vi "NMR10.vi"() -> ()   [LabVIEW 2013]
uses:
  <vilib>/Analysis/NI_AALBase.lvlib
panel:
  in  "Amp of Q curve":dbl=16.5 format="%_3f"
  in  "Subtract Q curve":bool=TRUE
  in  "Adjust Tune":bool=TRUE
  out "IF Offset":dbl(graph)=3.131691772460936
  out "Pedestal Difference":dbl(graph)=0.04542741927075716
  out "# Good Spectra":i32=99
  in  "Quality cuts":bool=TRUE
  out "Pedestal OK":bool=TRUE
  out "Sweep #":i32=2
  out "1st Sweep":bool
  out "ADC voltages OK":bool=TRUE
  out "Peak Height Distribution":cluster{"Y":dbl[], "Y":dbl[]}[](graph)=[{"Y"=[0.2355519843953429, 0.23617339654540798, 0.2367948086954731, 0.2374162208455382, 0.2380376329956033, 0.2386590451456684, 0.23928045729573352, 0.2399018694457986, 0.24052328159586372, 0.2411446937459288, 0.24176610589599393, 0.24238751804605904, 0.24300893019612413, 0.24363034234618924, 0.24425175449625433, 0.24487316664631945, 0.24549457879638456, 0.24611599094644965, 0.24673740309651476, 0.24735881524657988, 0.24798022739664496, 0.24860163954671008, 0.24922305169677517, 0.24984446384684028, 0.2504658759969054, 0.2510872881469705, 0.25170870029703557, 0.2523301124471007, 0.2529515245971658, 0.2535729367472309, 0.25419434889729603, 0.25481576104736114, 0.2554371731974262, 0.2560585853474913, 0.25667999749755643, 0.25730140964762155, 0.25792282179768666, 0.2585442339477517, 0.25916564609781684, 0.25978705824788195, 0.26040847039794707, 0.2610298825480122, 0.26165129469807724, 0.26227270684814236, 0.26289411899820747, 0.2635155311482726, 0.2641369432983377, 0.26475835544840276, 0.2653797675984679, 0.266001179748533, 0.2666225918985981, 0.2672440040486632, 0.26786541619872833, 0.2684868283487934, 0.2691082404988585, 0.2697296526489236, 0.27035106479898874, 0.27097247694905385, 0.2715938890991189, 0.272215301249184, 0.27283671339924914, 0.27345812554931426, 0.27407953769937937, 0.27470094984944443, 0.27532236199950955, 0.27594377414957466, 0.2765651862996398, 0.2771865984497049, 0.27780801059976995, 0.27842942274983506, 0.2790508348999002, 0.2796722470499653, 0.2802936592000304, 0.2809150713500955, 0.2815364835001606, 0.2821578956502257, 0.2827793078002908, 0.28340071995035593, 0.28402213210042104, 0.2846435442504861, 0.2852649564005512, 0.28588636855061633, 0.28650778070068145, 0.28712919285074656, 0.2877506050008116, 0.28837201715087674, 0.28899342930094185, 0.28961484145100697, 0.2902362536010721, 0.29085766575113714, 0.29147907790120225, 0.29210049005126737, 0.2927219022013325, 0.2933433143513976, 0.2939647265014627, 0.2945861386515278, 0.2952075508015929, 0.295828962951658, 0.2964503751017231, 0.29707178725178823], "Y"=[1.0, 0.0, 0.0, 0.0, 0.0, 0.0, 0.0, 0.0, 0.0, 0.0, 0.0, 1.0, 0.0, 0.0, 1.0, 0.0, 0.0, 0.0, 0.0, 0.0, 0.0, 0.0, 1.0, 1.0, 0.0, 1.0, 1.0, 2.0, 0.0, 1.0, 3.0, 1.0, 1.0, 0.0, 3.0, 2.0, 2.0, 2.0, 3.0, 2.0, 0.0, 4.0, 1.0, 1.0, 4.0, 3.0, 3.0, 2.0, 4.0, 0.0, 4.0, 2.0, 3.0, 1.0, 1.0, 2.0, 4.0, 4.0, 3.0, 0.0, 3.0, 4.0, 2.0, 2.0, 1.0, 2.0, 0.0, 1.0, 0.0, 0.0, 1.0, 2.0, 0.0, 0.0, 1.0, 1.0, 1.0, 0.0, 0.0, 1.0, 0.0, 0.0, 0.0, 0.0, 0.0, 1.0, 0.0, 0.0, 0.0, 0.0, 0.0, 0.0, 0.0, 0.0, 0.0, 0.0, 0.0, 0.0, 0.0, 1.0]}]
  in  "# of Sweeps":i32=100
  out "Std Dev (V)":dbl=0.009965193633611454 format="%_2g"
  out "Peak mean (V)":dbl=0.2655884316981644 format="%_4g"
  out "Peak Height":dbl(graph)=0.26806171289062286
  in  "Raw Data":bool
  in  "Tank RF ON":bool=TRUE
  in  "IF Atten (dB)":i8 min=0 max=35 step=5
  in  "IFoffset (V)":dbl=3.131691772460936 min=0.0 max=3000.0 step=0.001 format="%.3f"
  in  "Tune  (V)":dbl=1.5059999999999982 min=0.0 max=5.0 step=0.001 format="%.3f"
  in  "Hi / Lo Gain":bool
  out "Voltage Array":sgl[](array[numeric])=[0.39486083, 0.39415282, 0.37740478, 0.36463624, 0.35776368, 0.33198243, 0.3107544, 0.32425538, 0.2953125, 0.27941895, 0.2874756, 0.2617798, 0.2520508, 0.24379882, 0.24141845, 0.22194824, 0.19313964, 0.1977295, 0.19276123, 0.17390136, 0.17283936, 0.16755371, 0.14387207, 0.12849121, 0.12796631, 0.13111572, 0.1216919, 0.10755615, 0.08287354, 0.06949463, 0.07113037, 0.062060546, 0.036108397, 0.032678224, 0.013000488, 0.0095825195, 0.01607666, 0.0040771486, 0.005566406, -0.01229248, 0.0024536133, -0.0022338866, -0.017175293, -0.029064942, -0.02878418, -0.05206299, -0.04116211, -0.05924072, -0.060913086, -0.07078858, -0.06147461, -0.0708252, -0.09482422, -0.09287109, -0.08811035, -0.10527344, -0.10979004, -0.09885254, -0.10852051, -0.12213135, -0.12347412, -0.13558349, -0.13809815, -0.1430664, -0.16062012, -0.16202393, -0.16688232, -0.1687622, -0.1630371, -0.17376709, -0.19066162, -0.17672119, -0.19134521, -0.19102784, -0.20743409, -0.1963379, -0.19866943, -0.20877686, -0.2253662, -0.21699218, -0.22194824, -0.22015381, -0.22921142, -0.21680908, -0.21575928, -0.23323974, -0.21798095, -0.22463378, -0.23702392, -0.21989746, -0.22541504, -0.20744629, -0.202063, -0.19719239, -0.18527833, -0.18197021, -0.13729247, -0.11975098, -0.061206054, -0.022375489, 0.010229493, 0.036230467, -0.003857422, -0.054382324, -0.0927124, -0.12541504, -0.1385376, -0.15421143, -0.16003418, -0.15662841, -0.19451904, -0.18380126, -0.19353028, -0.19848633, -0.19445801, -0.21176758, -0.20693359, -0.19925538, -0.19172363, -0.18999024, -0.19869384, -0.18461914, -0.19050293, -0.18470459, -0.18983154, -0.1901001, -0.20270996, -0.18931885, -0.18898925, -0.16983643, -0.17060547, -0.16373292, -0.16271973, -0.16048583, -0.1584961, -0.1397461, -0.14522704, -0.1364624, -0.13929443, -0.13120118, -0.11820068, -0.09746094, -0.105810545, -0.11616211, -0.11202393, -0.0831543, -0.08693848, -0.07366943, -0.076123044, -0.06868897, -0.05710449, -0.052990723, -0.0430542, -0.017224122, -0.010522461, -0.02224121, 0.0063842773, 0.0071655274, 0.009472656, 0.024536133, 0.02734375, 0.017590333, 0.036035158, 0.04018555, 0.06090088, 0.066381834, 0.084106445, 0.078625485, 0.09157715, 0.09299316, 0.107104495, 0.11695556, 0.118334964, 0.1282959, 0.134375, 0.17685547, 0.15549317, 0.17213134, 0.19041748, 0.2119873, 0.21591797, 0.22495118, 0.23574218, 0.23773193, 0.2640869, 0.2647583, 0.27943116, 0.28809816, 0.30527344, 0.32390136, 0.32923585, 0.334021, 0.34277344, 0.3604126, 0.37745363, 0.3977661, 0.40411377, 0.4104004, 0.42994386, 0.43033448, 0.4552002] format="%.4f"
  in  "Invert Polarity":bool=TRUE
  out "NMR Spectrum":cluster{dbl, "Step Width (MHz)":dbl, dbl[]}(graph)={224.59, "Step Width (MHz)"=0.002, [-0.03990791601558322, -0.02741592382802091, -0.031095970703144654, -0.030928525390583078, -0.024997083984272722, -0.038106333984392754, -0.04679436132808315, -0.02088538476552451, -0.03755225585939084, -0.041301810546833156, -0.0212331699217764, -0.03504897070313909, -0.03302997460933313, -0.02966592773427859, -0.020562298828137343, -0.028680513671833358, -0.046269107421780614, -0.03059126367188572, -0.024603525390583664, -0.032639388671782815, -0.023009400390634233, -0.01773504492183406, -0.03098868554678516, -0.03607354492188283, -0.026434447265584554, -0.013253033203037473, -0.012776861328131467, -0.017144603515585083, -0.03219122070303995, -0.03606612695313019, -0.025058384765585667, -0.02488820898429253, -0.04173235742187906, -0.036186533203086485, -0.0470202675780452, -0.04172623632812797, -0.026652095703087325, -0.030203607421797868, -0.020398349609377003, -0.030073236328088254, -0.007275142578050731, -0.004042642578126088, -0.01119604882808925, -0.015429697265553627, -0.007624935546875294, -0.023511744140590346, -0.005350865234306668, -0.01630147851562458, -0.010977841796841525, -0.013989330078059775, 0.0020566347656260364, -0.0006939511718428437, -0.018224974609312966, -0.00993584960937341, 0.0010288925781558045, -0.010062193359316213, -0.008638794921872944, 0.008106705078154336, 0.004114736328180407, -0.0039521035156226125, 0.00011712304690278397, -0.00671225195307304, -0.004078900390622364, -0.004031162109348868, -0.016700873046895076, -0.0133526816406222, -0.013591080078100587, -0.010982962890643072, -0.0009018652343721067, -0.007407845703102406, -0.02021037695314118, -0.002309947265622142, -0.01310597070310432, -0.009092587890639381, -0.0219348378906222, -0.007406646484356322, -0.006438189453137649, -0.013377611328122402, -0.02693096679685844, -0.015652943359386023, -0.017836998046872693, -0.01340256445311061, -0.019952181640634475, -0.005173837890623034, -0.0018800332031128908, -0.017248501953133044, -9.712890623514436e-06, -0.004814544921865255, -0.01548868164063169, 0.0032217832031259386, -0.0008437949218676744, 0.01844495507811958, 0.025016255859375308, 0.03094286132812976, 0.043780923828120766, 0.04788102929687457, 0.09321876367187712, 0.11128826757812185, 0.17022918945312376, 0.2093237558593744, 0.24206073632812286, 0.26806171289062286, 0.22784182226562158, 0.17705291992187377, 0.13832684179687185, 0.10509620507811868, 0.09131364648437457, 0.07484781835937077, 0.0681010644531157, 0.07045082617187531, 0.03137220117186959, 0.0407699746093626, 0.02958897070312594, 0.023048916015618315, 0.025361236328109438, 0.006203666015626497, 0.009057650390616956, 0.014623873046856167, 0.019911611328126966, 0.01926900976561549, 0.008057396484352802, 0.0194921035156273, 0.010836314453113977, 0.013730654296849387, 0.005567701171877604, 0.002131146484362356, -0.01377871679690415, -0.003819603515622244, -0.007054013671889375, 0.008402818359342229, 0.0038057753906279024, 0.00671833398435881, 0.0036395175780885025, 0.0016494042968778766, -0.0007168496093930832, 0.01354515039058471, 0.0034441933593777896, 0.007456841796854935, -0.0002591894531691896, 0.002818072265627636, 0.010670560546852864, 0.026130306640576834, 0.012368697265627365, -0.0035268652343992957, -0.0050646816406772766, 0.017996947265627034, 0.008272767578098417, 0.015469810546818591, 0.006812197265626568, 0.007910279296846096, 0.013026751953064325, 0.010540521484376036, 0.013745044921843641, 0.03271112304680998, 0.03241678320312541, 0.013570033203091109, 0.03493552148430554, 0.028324771484374706, 0.023107900390588493, 0.030515376953051038, 0.025534994140623907, 0.007861576171835777, 0.018254400390546405, 0.014220791015623013, 0.026620123046833005, 0.023653080078041733, 0.03279768945312203, 0.018604732421830056, 0.022712392578036866, 0.015152408203120915, 0.02015573632807713, 0.020766810546782005, 0.012774205078119799, 0.013231142578074034, 0.009674244140527088, 0.042386712890618516, 0.011124408203070868, 0.01773059179677197, 0.02585272460936719, 0.037126548828067624, 0.030629212890516844, 0.02910241601561575, 0.029201431640564324, 0.020367177734261582, 0.03576615820311427, 0.02534954492181088, 0.028802396484256226, 0.026117388671862612, 0.03180868164055736, 0.03882061132816686, 0.0324070839843609, 0.025312240234303757, 0.022052681640666844, 0.02754784179685918, 0.03231285742180004, 0.04021735742191687, 0.03402501367185726, 0.027639634765546178, 0.03437909179691692, 0.02183371679685539, 0.03363143945304234]}
  out "Pedestal Diff (V)":sgl=0.04542742 format="%.3f"
  out "Peak amp (V)":sgl=0.26806173 format="%.3f"
  in  "Save Data to File":bool
  in  "RF Level (dBm)":dbl=-2.0000000000000004 min=-10.0 max=1.0 step=0.1 format="%.2f"
  out "SMT error out":errorcluster
  out "Sample RMS  (V)":dbl=0.014719094355728133 format="%.4f"
  in  "# Sample/step":i32=100 min=1 max=1000 step=100
  in  "ADC Rate (Hz)":i32=10000 min=1 max=20000 step=1000
  in  "ADC Range":i32(ring)=1 items=["+- 10 V"=1, "+- 2.5 V"=3]
  in  "Step Width (MHz)":dbl=0.002 min=0.0 max=1000.0 step=0.0005 format="%.4f"
  in  "Freq Span (MHz)":dbl=0.4 min=0.0 max=3000.0 step=0.1 format="%.3f"
  in  "Center Freq (MHz)":dbl=224.79 min=0.005 max=6000.0 step=0.1 format="%.3f"
  in  "Sweep Mode":u16(ring)=3 items=["Off", "Single", "Auto", "Step"]
  in  "GPIB Addr (28)":refnum<visa-resource-name>="GPIB0::28::INSTR"
  # "E1039 Prototype NMR Control Panel"
  # "Settings"
  # "D\nA\nC"
  # "R\nF\n\nG\ne\nn\ne\nr\na\nt\no\nr"
  # "A\nD\nC"
  # "D\na\nt\na"
  # "I\n/\nO"
  # "Results"
  # "A\nv\ne\nr\na\ng\ne"
  # "S\nw\ne\ne\np"
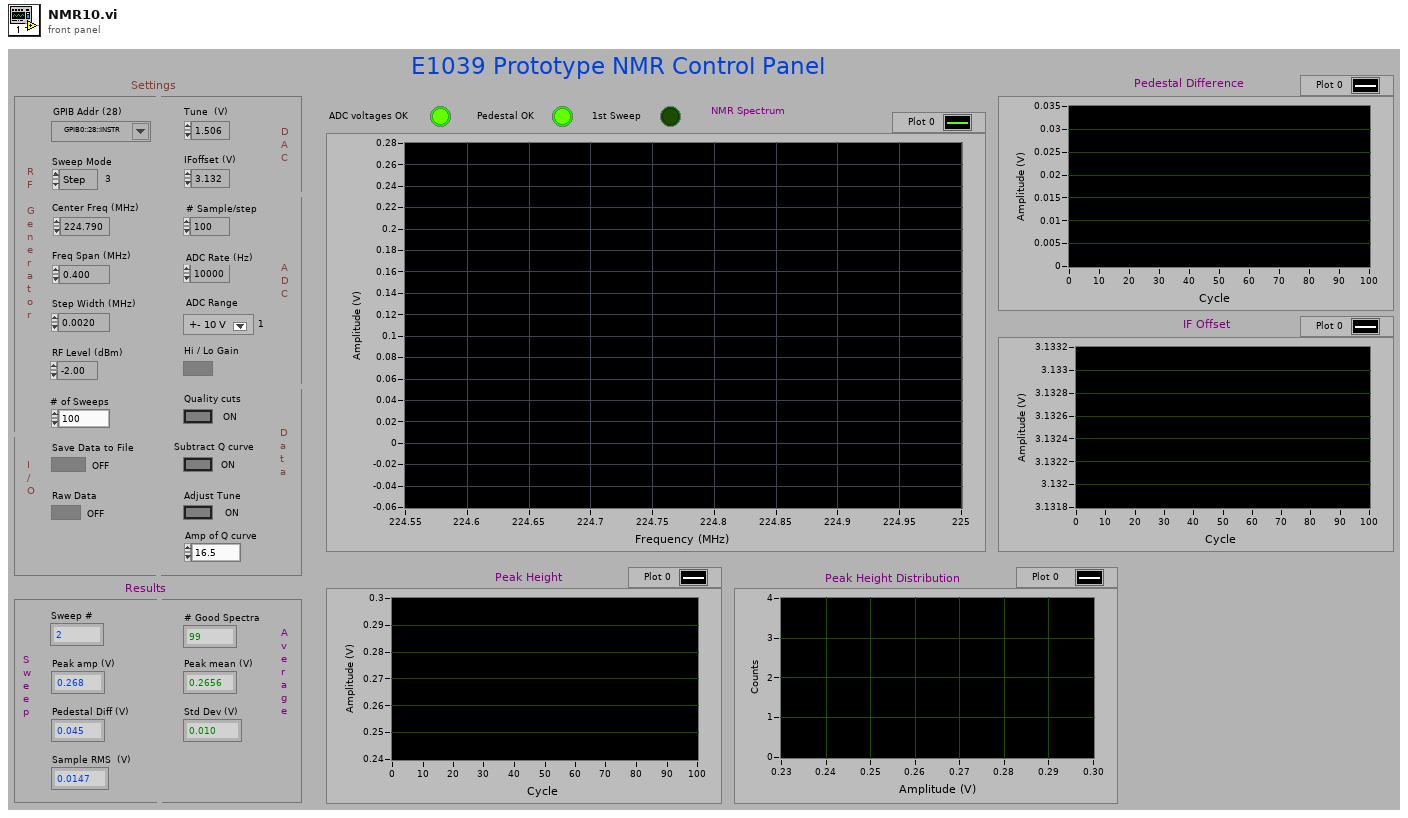
[diagram p1: front panel]
types:
  T1 = cluster{dbl, "Step Width (MHz)":dbl, "Corrected data":dbl[]}
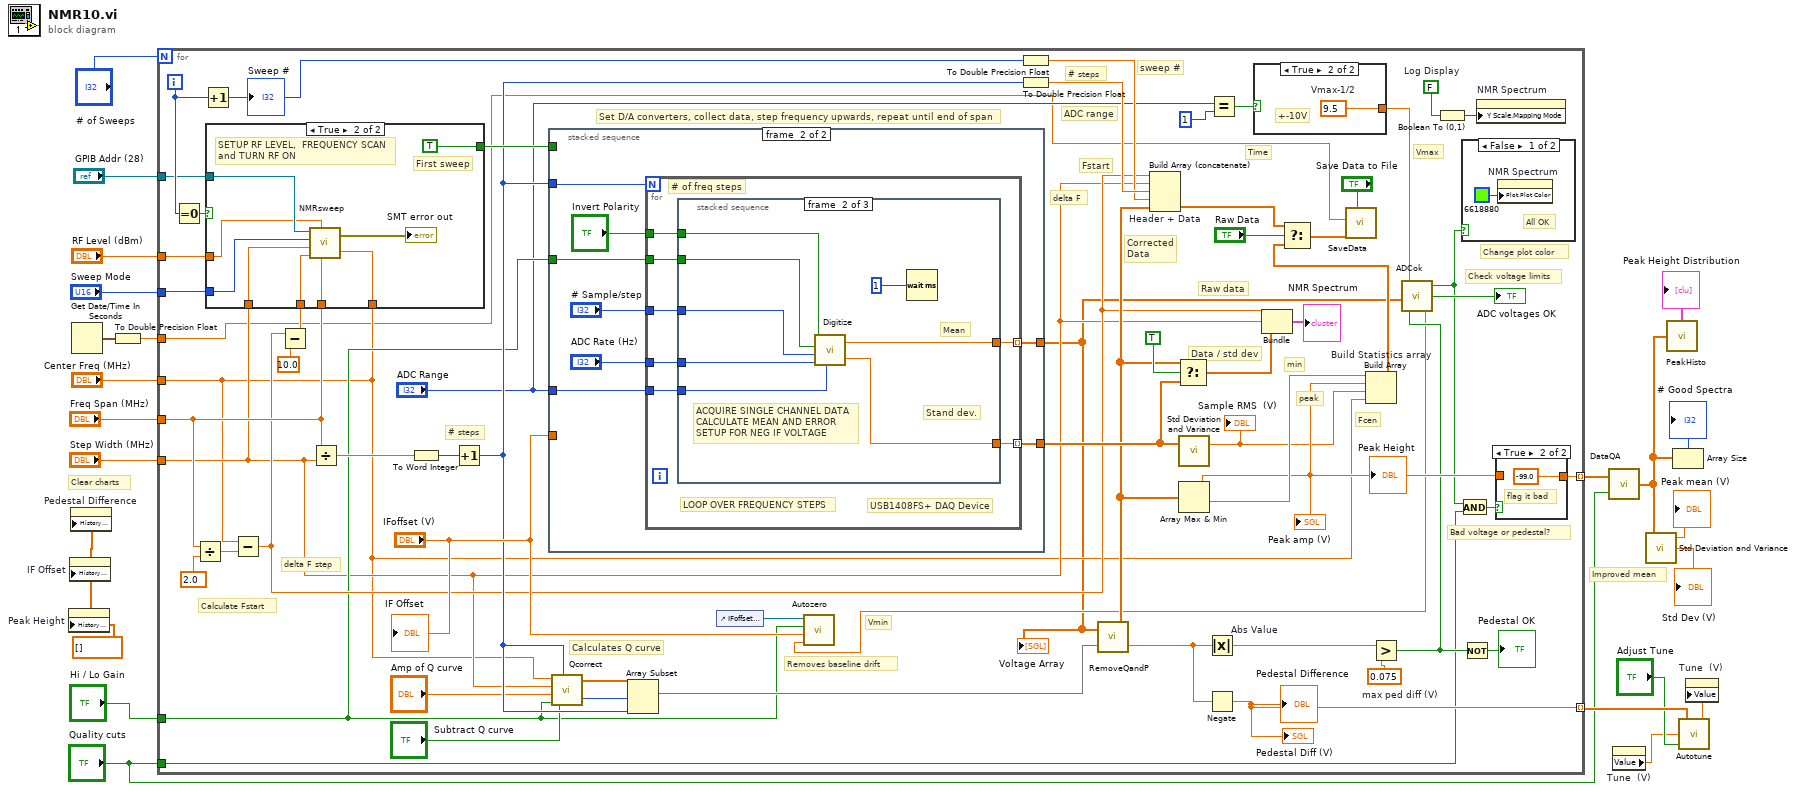
[diagram p0: block diagram]
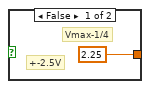
[diagram p2: hidden frame]
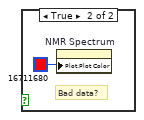
[diagram p3: hidden frame]
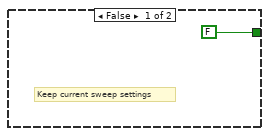
[diagram p5: hidden frame]
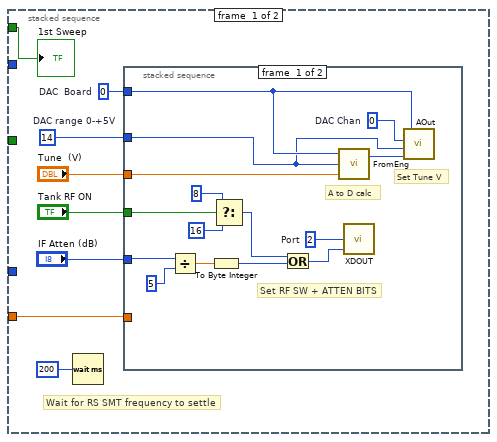
[diagram p6: hidden frame]
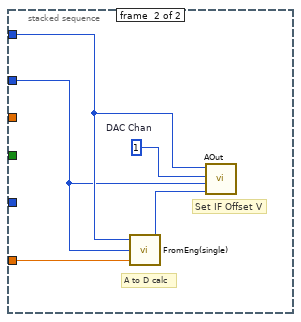
[diagram p7: hidden frame]
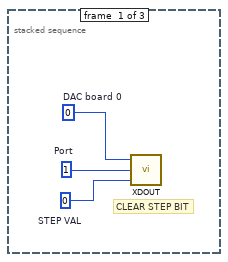
[diagram p8: hidden frame]
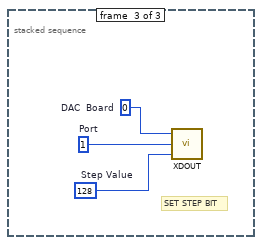
[diagram p9: hidden frame]
diagram:
  w6 = dbl[] []
  # "Clear charts"
  # "Improved mean"
  n1 = property on="Peak Height" class="WFChart (strict)"("History Data"=w6) -> ()  [unwired: 2 in, 2 out]
  n2 = property on="IF Offset" class="WFChart (strict)"("History Data"=w6) -> ()  [unwired: 2 in, 2 out]
  n3 = property on="Pedestal Difference" class="WFChart (strict)"("History Data"=w6) -> ()  [unwired: 2 in, 2 out]
  n4 = Get Date/Time In Seconds() -> (seconds since 1Jan1904=w2:timestamp)
  n5 = To Double Precision Float(number=w2) -> (double precision float=w1:dbl)
  n6 = for {
    N: "# of Sweeps" -> [_]
    tunnel: [w62] -> w18 mode=indexing
    tunnel: "Quality cuts" -> [w31]
    tunnel: [w40] -> w15 mode=indexing
    tunnel: "Center Freq (MHz)" -> [w27]
    tunnel: "Freq Span (MHz)" -> [w46]
    tunnel: "Step Width (MHz)" -> [w29]
    tunnel: "Sweep Mode" -> [w44]
    tunnel: "Hi / Lo Gain" -> [w43]
    tunnel: "GPIB Addr (28)" -> [w42]
    tunnel: "RF Level (dBm)" -> [w41]
    tunnel: w1 -> [w23]
    i -> [w59]
    w80 = FALSE  # Log Display
    w63 = 0.075  # max ped diff (V)
    # "Time"
    # "Vmin"
    # "min"
    # "peak"
    # "Raw data"
    # "Corrected\nData"
    # "Fstart"
    # "delta F"
    # "# steps"
    # "ADC range"
    # "sweep #"
    # "Fcen"
    # "Set D/A converters, collect data, step frequency upwards, repeat until end of span"
    # "Vmax"
    # "Calculates Q curve"
    # "Removes baseline drift"
    # "Change plot color"
    # "Bad voltage or pedestal?"
    # "Check voltage limits"
    # "Data / std dev"
    # "# steps"
    # "Calculate Fstart"
    # "delta F step"
    n7 = Equal To 0?(x=w59) -> (x = 0?=w65:bool)
    n8 = Divide(x=w46, y=sgl 2.0) -> (x/y=w81:dbl)
    n9 = Increment(x=w59) -> (x+1=w49:i32)
    "Sweep #" <- w49
    n10 = Subtract(x=w27, y=w81) -> (x-y=w45:dbl)
    n11 = Subtract(x=w45, y=10.0) -> (x-y=w76:dbl)
    n12 = case shown="True" w65 {
      tunnel: w76 -> [_ w99]
      tunnel: w29 -> [_ w97]
      tunnel: w27 -> [_ w96]
      tunnel: w46 -> [_ w98]
      tunnel: [FALSE TRUE] -> w64
      tunnel: w44 -> [_ w93]
      tunnel: w42 -> [_ w92]
      tunnel: w41 -> [_ w91]
      frame False {
        # "Keep current sweep settings"
      }
      frame True {
        # "First sweep"
        # "SETUP RF LEVEL,  FREQUENCY SCAN\nand TURN RF ON"
        n13 = call "NMRsweep.vi"("Center Freq (MHz)"=w96, "Freq Span (MHz)"=w98, "RF Level (dBm)"=w91, "Foffset (MHz)"=w99, "Step Width (MHz)"=w97, "Sweep Mode"=w93, "GPIB Addr (28)"=w92) -> ("error out"=→"SMT error out":errorcluster)
      }
    }
    n14 = Divide(x=w46, y=w29) -> (x/y=w83:dbl)
    n15 = To Word Integer(number=w83) -> (16bit integer=w77:i16)
    n16 = Increment(x=w77) -> (x+1=w53:i16)
    n17 = stacked-sequence {
      tunnel: [_ w135] -> w68
      tunnel: [_ w134] -> w26
      tunnel: w53 -> [_ w133]
      tunnel: "IFoffset (V)" -> [w101 _]
      tunnel: w43 -> [_ w132]
      tunnel: w64 -> [w100 _]
      tunnel: "ADC Range" -> [_ w131]
      frame #0 {
        w105 = 14  # DAC range 0-+5V
        w106 = 0  # DAC  Board
        # "Wait for RS SMT frequency to settle"
        n18 = Wait (ms)(milliseconds to wait=200) -> ()  [unwired: 1 out]
        n19 = stacked-sequence {
          tunnel: w106 -> [w113 w125]
          tunnel: w105 -> [w112 w124]
          tunnel: "Tune  (V)" -> [w111 _]
          tunnel: "Tank RF ON" -> [w109 _]
          tunnel: "IF Atten (dB)" -> [w108 _]
          tunnel: w101 -> [_ w123]
          frame #0 {
            w115 = 2  # Port
            w122 = 0  # DAC Chan
            # "A to D calc"
            # "Set RF SW + ATTEN BITS"
            # "Set Tune V"
            n20 = Divide(x=w108, y=5) -> (x/y=w120:dbl)
            n21 = To Byte Integer(number=w120) -> (8bit integer=w117:i8)
            n22 = Select(t=8, s=w109, f=16) -> (s? t:f=w116:i32)
            n23 = Or(x=w116, y=w117) -> (x .or. y?=w114:i32)
            n24 = call-poly "FromEng.VI"("Eng Units"=w111, "Range"=w112, "BoardNum (0)"=w113) -> ("DA Data"=w110:u16)  [unwired: 1 out]
            n25 = call "XDOUT.VI"(2:w114, "PortNum"=w115) -> ()  [unwired: 3 in]
            n26 = call "AOut.VI"("DataValue"=w110, "Range"=w112, "Channel"=w122, "BoardNum"=w113) -> ()  [unwired: 1 out]
          }
          frame #1 {
            w127 = 1  # DAC Chan
            # "A to D calc"
            # "Set IF Offset V"
            n27 = call "FromEng(single).VI"("Eng Units"=w123, "Range"=w124, "BoardNum (0)"=w125) -> ("DA Data"=w126:u16)  [unwired: 1 out]
            n28 = call "AOut.VI"("DataValue"=w126, "Range"=w124, "Channel"=w127, "BoardNum"=w125) -> ()  [unwired: 1 out]
          }
        }
        "1st Sweep" <- w100
      }
      frame #1 {
        n29 = for {
          N: w133 -> [_]
          tunnel: [w142] -> w134 mode=indexing
          tunnel: [w141] -> w135 mode=indexing
          tunnel: w132 -> [w140]
          tunnel: w131 -> [w139]
          tunnel: "ADC Rate (Hz)" -> [w138]
          tunnel: "# Sample/step" -> [w137]
          tunnel: "Invert Polarity" -> [w136]
          # "# of freq steps"
          # "USB1408FS+ DAQ Device"
          # "LOOP OVER FREQUENCY STEPS"
          n30 = stacked-sequence {
            tunnel: [_ w152 _] -> w142
            tunnel: [_ w151 _] -> w141
            tunnel: w140 -> [_ w150 _]
            tunnel: w139 -> [_ w149 _]
            tunnel: w138 -> [_ w148 _]
            tunnel: w137 -> [_ w147 _]
            tunnel: w136 -> [_ w146 _]
            frame #0 {
              w143 = 0  # DAC board 0
              w144 = 0  # STEP VAL
              w145 = 1  # Port
              # "CLEAR STEP BIT"
              n31 = call "XDOUT.VI"(2:w144, "PortNum"=w145, "BoardNum"=w143) -> ()  [unwired: 2 in]
            }
            frame #1 {
              # "Stand dev."
              # "Mean"
              # "ACQUIRE SINGLE CHANNEL DATA\nCALCULATE MEAN AND ERROR\nSETUP FOR NEG IF VOLTAGE"
              n32 = call "Digitize.vi"("Invert Polarity"=w146, "IF or Log"=w150, "# Sample/step"=w147, "ADC Rate (Hz)"=w148, "ADC Range"=w149) -> ("mean"=w152:dbl, "standard deviation"=w151:dbl)
              n33 = Wait (ms)(milliseconds to wait=1) -> ()  [unwired: 1 out]
            }
            frame #2 {
              w154 = 128  # Step Value
              w156 = 0  # DAC  Board
              w155 = 1  # Port
              # "SET STEP BIT"
              n34 = call "XDOUT.VI"(2:w154, "PortNum"=w155, "BoardNum"=w156) -> ()  [unwired: 2 in]
            }
          }
        }
      }
    }
    "Voltage Array" <- w26
    n35 = call "Qcorrect.vi"("Subtract Q curve"="Subtract Q curve", "Nstep"=w53, "IF or Log"=w43, "Amp of Q curve"="Amp of Q curve", "Step Width (MHz)"=w29, "Center Freq (MHz)"=w27) -> ("Start"=w70:i32, "Array"=w71:dbl[])
    n36 = Array Subset "Array Subset"(array=w71, index=w70, length=w53) -> (w69:dbl[])
    n37 = control-ref of="IFoffset (V)"() -> (w34:refnum<vi>)
    n38 = To Double Precision Float(number=w49) -> (double precision float=w50:dbl)
    n39 = To Double Precision Float(number=w53) -> (double precision float=w52:dbl)
    n40 = call "RemoveQandP.vi"("Qcurve"=w69, "Raw data"=w26) -> ("Ped L-R"=w55:dbl, "Corrected data"=w51:dbl[])
    n41 = Build Array (concatenate) "Header + Data"(w45, w29, w52, w50, w51) -> (w54:dbl[])
    n42 = Select(t=w51, s=TRUE, f=w68) -> (s? t:f=w73:dbl[])
    n43 = call <vilib>:"Std Deviation and Variance.vi"("X"=w68) -> ("mean"=w28:dbl)  [unwired: 1 in, 2 out]
    "Sample RMS  (V)" <- w28
    n44 = Array Max & Min(array=w51) -> (max value=w61:dbl, min value=w67:dbl)  [unwired: 2 out]
    "Peak amp (V)" <- w61
    "Peak Height" <- w61
    n45 = Absolute Value "Abs Value"(x=w55) -> (abs(x)=w57:dbl)
    n46 = Negate(x=w55) -> (-x=w40:dbl)
    "Pedestal Diff (V)" <- w40
    "Pedestal Difference" <- w40
    n47 = Equal?(x="ADC Range", y=1) -> (x = y?=w38:bool)
    n48 = case shown="True" w38 {
      tunnel: [2.25 w85] -> w35
      frame False {
        # "Vmax-1/4"
        # "+-2.5V"
      }
      frame True {
        w85 = 9.5  # Vmax-1/2
        # "+-10V"
      }
    }
    n49 = Bundle(w45, "Step Width (MHz)"=w29, "Corrected data"=w73) -> (→"NMR Spectrum":T1)  [unwired: 1 in]
    n50 = Build Array "Build Statistics array"(w67, w61, w28, w27) -> (w75:dbl[])
    n51 = Select(t=w54, s="Raw Data", f=w75) -> (s? t:f=w24:dbl[])
    n52 = call "SaveData.vi"("Array"=w24, "Save Data to File"="Save Data to File", "Ext time (sec)"=w23) -> ()  [unwired: 1 out]
    n53 = Greater?(x=w57, y=w63) -> (0:w39:bool)
    n54 = call "ADCok.vi"("PedOK"=w39, "Array"=w26, "Vmax-1/2"=w35) -> ("Vmin"=w33:dbl, "ADC voltages OK"=→"ADC voltages OK":bool, "Allok"=w30:bool)
    n55 = call "Autozero.vi"("Vmin (V)"=w33, "IFoffset (V)"="IFoffset (V)", "IF or Log"=w43, "reference"=w34) -> ()
    n56 = Boolean To (0,1)(Boolean=w80) -> (0, 1=w78:i16)
    n57 = And(x=w30, y=w31) -> (x .and. y?=w58:bool)
    n58 = case shown="False" w30 {
      frame False {
        # "All OK"
        n59 = property on="NMR Spectrum" class="WFGraph (strict)"("Plot.Plot Color"=u32 6618880) -> ()  [unwired: 2 in, 2 out]
      }
      frame True {
        # "Bad data?"
        n60 = property on="NMR Spectrum" class="WFGraph (strict)"("Plot.Plot Color"=u32 16711680) -> ()  [unwired: 2 in, 2 out]
      }
    }
    n61 = Not(x=w39) -> (.not. x?=→"Pedestal OK":bool)
    n62 = property on="NMR Spectrum" class="WFGraph (strict)"("Y Scale.Mapping Mode"=w78) -> ()  [unwired: 2 in, 2 out]
    n63 = case shown="True" w58 {
      tunnel: [w88 -99.0] -> w62
      tunnel: w61 -> [w88 _]
      frame False {
        # "Data OK"
      }
      frame True {
        # "flag it bad"
      }
    }
    "IF Offset" <- "IFoffset (V)"
  }
  n64 = call "DataQA.vi"("Quality cuts"="Quality cuts", "Data In"=w18) -> ("Data Out"=w17:dbl[])
  n65 = property on="Tune  (V)" class="DigNum (strict)"() -> ("Value"=w5:dbl)  [unwired: 2 in, 2 out]
  n66 = call <vilib>:"Std Deviation and Variance.vi"("X"=w17) -> ("mean"=→"Peak mean (V)":dbl, "standard deviation"=→"Std Dev (V)":dbl)  [unwired: 1 in, 1 out]
  n67 = call "PeakHisto.vi"("Data Out"=w17) -> ("XY Graph"=→"Peak Height Distribution":cluster{"Y":dbl[], "Y":dbl[]}[])
  n68 = Array Size(array=w17) -> (size(s)=→"# Good Spectra":i32)
  n69 = call "Autotune.vi"("Adjust Tune"="Adjust Tune", "Tune Vin"=w5, "Pedestal Diff"=w15) -> ("Tune Vout"=w4:dbl)
  n70 = property on="Tune  (V)" class="DigNum (strict)"("Value"=w4) -> ()  [unwired: 2 in, 2 out]
